vi "Read Pie Position.vi"(8 "error in (no error)":errorcluster, 11 "Data Value Reference in":refnum<data-value>) -> (0 "error out":errorcluster, 2 "Slice Positions":T1)   [LabVIEW 2018, in "PieChart.lvclass"]
uses:
  PieChart.lvclass
  <vilib>/Utility/miscctls.llb/LVFontTypeDef.ctl
  State Data.ctl
  <vilib>/Utility/miscctls.llb/LVBoundsTypeDef.ctl
  Pie info for Click.ctl
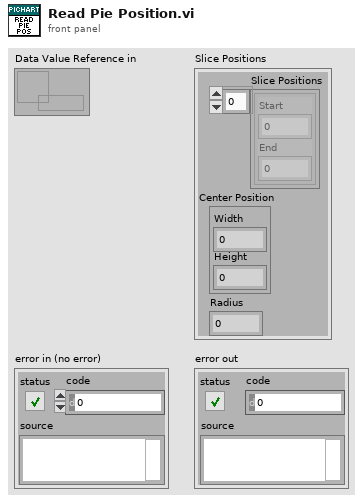
[diagram p1: front panel]
types:
  T1 = typedef "PieChart.lvclass/Pie info for Click.ctl" = cluster{"Slice Positions":cluster{"Start":i16, "End":i16}[], "Center Position":T2, "Radius":i16}
  T2 = typedef "LVBoundsTypeDef.ctl" = cluster{"Width":u32, "Height":u32}
  T3 = typedef "PieChart.lvclass/State Data.ctl" = cluster{"Title":string, "Values[]":dbl[], "Labels[]":string[], "Colors[]":u32[], "Include Legend?":bool, "Include Title?":bool, "Title Font":T4, "Legend Font":T4, "Selection":i32, "Slice Positions":T1}
  T4 = typedef "LVFontTypeDef.ctl" = cluster{"Font Name":string, "Size":u16, "Bold":bool, "Italic":bool, "Underline":bool, "Strikeout":bool, "Color":u32}
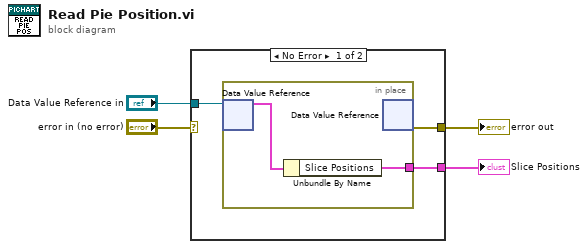
[diagram p0: block diagram]
diagram:
  n1 = case shown="No Error" "error in (no error)" {
    selector: "error in (no error)" -> [_ w10]
    tunnel: "Data Value Reference in" -> [w7 _]
    tunnel: [w6 w10] -> w3
    tunnel: [w5 _] -> w1
    frame No Error {
      n2 = in-place {
        in-place-border: [w8] -> w5
        n3 = in-place-dvr #1(w7) -> (w9:T3)  [unwired: 1 out]
        n4 = Unbundle By Name(w9) -> ("Slice Positions"=w8:T1)
        n5 = in-place-dvr #1() -> (w6:errorcluster)  [unwired: 1 in, 1 out]
      }
    }
    frame Error {
    }
  }
  "error out" <- w3
  "Slice Positions" <- w1
